vi "LWXPS_GroupMoveAbortFast.vi"(8 "LabVIEW error IN":errorcluster, 9 "Acceleration Multiplier":i32, 10 "Group Name":string, 11 "XPS Reference IN":refnum<k24>) -> (0 "LabVIEW error OUT":errorcluster, 1 "XPS Error String":string, 2 "Returned error code":i32, 3 "XPS Reference OUT":refnum<k24>)   [LabVIEW 2014]
uses:
  D:/XPSQ8_LabView_Library/Development/Source/Dll/Newport.XPS.CommandInterface.dll
  Dll/Newport.XPS.CommandInterface.dll
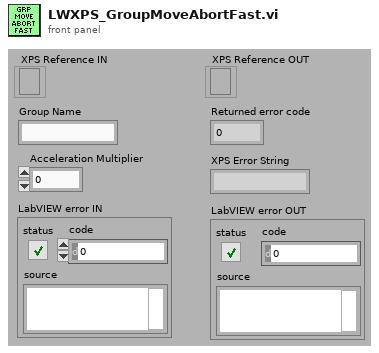
[diagram p1: front panel]
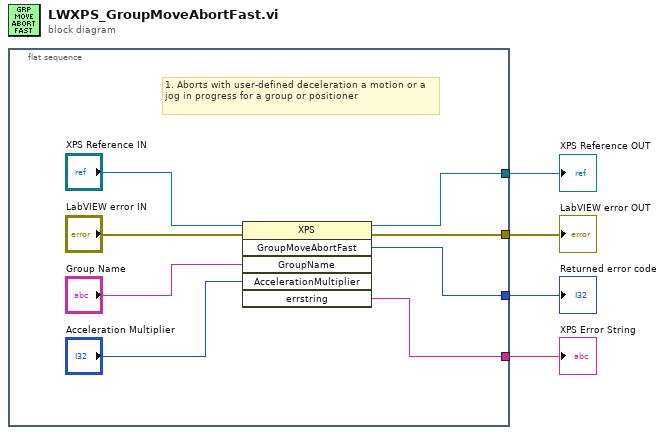
[diagram p0: block diagram]
diagram:
  n1 = flat-sequence {
    tunnel: [w10] -> w4
    tunnel: [w7] -> w3
    tunnel: [w11] -> w2
    tunnel: [w6] -> w1
    frame #0 {
      # "1. Aborts with user-defined deceleration a motion or a jog in progress for a group or positioner"
      n2 = invoke class="XPS" method="GroupMoveAbortFast"(reference="XPS Reference IN", error in="LabVIEW error IN", "GroupName"="Group Name", "AccelerationMultiplier"="Acceleration Multiplier") -> (reference out=w10:refnum<k24>, error out=w7:errorcluster, "GroupMoveAbortFast"=w11:i32, "errstring"=w6:string)  [unwired: 2 in, 2 out]
    }
  }
  "XPS Reference OUT" <- w4
  "LabVIEW error OUT" <- w3
  "Returned error code" <- w2
  "XPS Error String" <- w1
